vi "Conv_Rotations_Radians.vi"(10 "Rotations":dbl) -> (2 "Radians":dbl)   [LabVIEW 2019, in "Trajectory_Library.lvlib"]
doc: "Convert Rotations to Radians"
uses:
  Trajectory_Library.lvlib
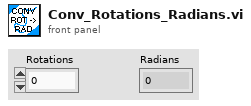
[diagram p1: front panel]
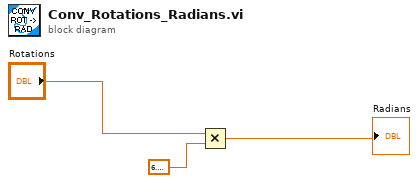
[diagram p0: block diagram]
diagram:
  n1 = Multiply(x="Rotations", y=6.283185307179586) -> (x*y=→"Radians":dbl)
